vi "Database_CloseConnection.vi"(2 "error in":errorcluster, 3 "connection reference":T1) -> (0 "error out":errorcluster)   [LabVIEW 2015]
uses:
  <vilib>/addons/database/Connection.llb/Conn ObjectReference.ctl
  <vilib>/addons/database/NI_Database_API.lvlib
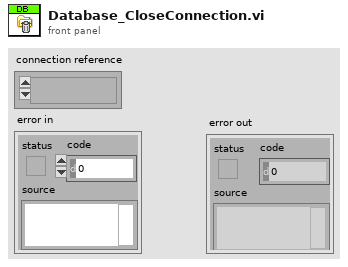
[diagram p1: front panel]
types:
  T1 = typedef "NI_Database_API.lvlib/Conn ObjectReference.ctl" = refnum<k1>
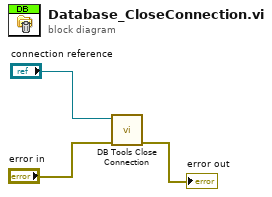
[diagram p0: block diagram]
diagram:
  n1 = call <vilib>:"DB Tools Close Connection.vi"("error in (no error)"="error in", "connection reference"="connection reference") -> ("error out"=→"error out":errorcluster)  [unwired: 5 in]
